vi "Stage1.vi"(10 "On?":bool, 11 "Stage 1 Speed":dbl) -> ()   [LabVIEW 2011]
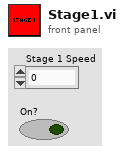
[diagram p1: front panel]
types:
  T1 = typedef "WPI_MotorControlDeviceRef.ctl" = cluster{"DeviceStatus":errorcluster, "Type":enum16{"PWM", "CAN"}, "PWM":cluster{"Digital Module":T2, "PWM Channel":T3, "DeadBand":T4}, "CAN":cluster{"Device Number":u8, "Control Mode":T5, "Semaphore":T6, "Max Vout":dbl}, "Invert":bool, "TransformRef":T7, "InvTransformRef":T7}
  T2 = typedef "FPGA_TypedefDigitalModule.ctl" = enum16{"Digital Module 1", "Digital Module 2"}
  T3 = typedef "FPGA_DIOPWMChannel.ctl" = enum8{"PWM 1", "PWM 2", "PWM 3", "PWM 4", "PWM 5", "PWM 6", "PWM 7", "PWM 8", "PWM 9", "PWM 10", "Invalid"}
  T4 = typedef "WPI_PWMDeadband.ctl" = cluster{"Name":string, "maxPositivePwm":i32, "minPositivePwm":i32, "centerPwm":i32, "maxNegativePwm":i32, "minNegativePwm":i32, "angularRange":u16}
  T5 = typedef "WPI_CANJaguar_ControlMode.ctl" = enum8{"Percent VBus", "Current", "Speed", "Position", "Voltage"}
  T6 = typedef "Semaphore RefNum" = refnum<k1>
  T7 = typedef "WPI_PWMTransform_ConPane.ctl" = refnum<vi>
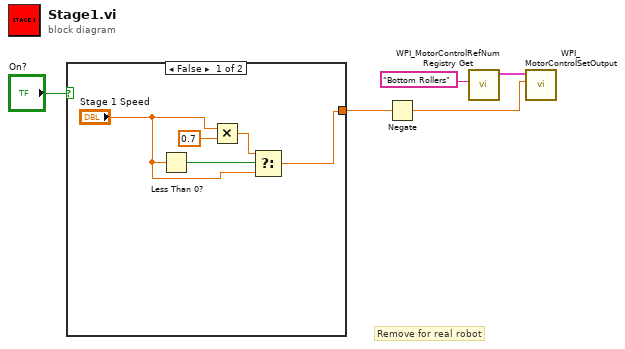
[diagram p0: block diagram]
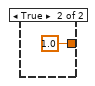
[diagram p2: hidden frame]
diagram:
  # "Remove for real robot"
  n1 = case shown="False" "On?" {
    tunnel: [w6 1.0 ("Bottom Speed")] -> w2
    frame False {
      n2 = Less Than 0?(x="Stage 1 Speed") -> (x < 0?=w8:bool)
      n3 = Multiply(x="Stage 1 Speed", y=0.7) -> (x*y=w9:dbl)
      n4 = Select(t=w9, s=w8, f="Stage 1 Speed") -> (s? t:f=w6:dbl)
    }
    frame True {
    }
  }
  n5 = Negate(x=w2) -> (-x=w1:dbl)
  n6 = call <vilib>:"WPI_MotorControlRefNum Registry Get.vi"("refnum name"="Bottom Rollers") -> ("MotorControlDevRef"=w4:T1)  [unwired: 9 in, 1 out]
  n7 = call <vilib>:"WPI_MotorControlSetOutput.vi"("Output"=w1, "MotorControlDevRef"=w4) -> ()  [unwired: 8 in, 2 out]
